vi "GetBarStartPosition.vi"(8 "error in (no error)":errorcluster, 11 "Code39 in":refnum<class "Code39.lvclass">) -> (0 "error out":errorcluster, 2 "Start Position":cluster{"x":i16, "y":i16}={"x"=10, "y"=3}, 3 "Code39 out":refnum<class "Code39.lvclass">)   [LabVIEW 2013, in "BarCodes.lvlib" / "Code39.lvclass"]
doc: "Specifies the top-left corner of the barcode in a given image. This effectively sets the quiet space in either direction around the bar code."
uses:
  Code39.lvclass
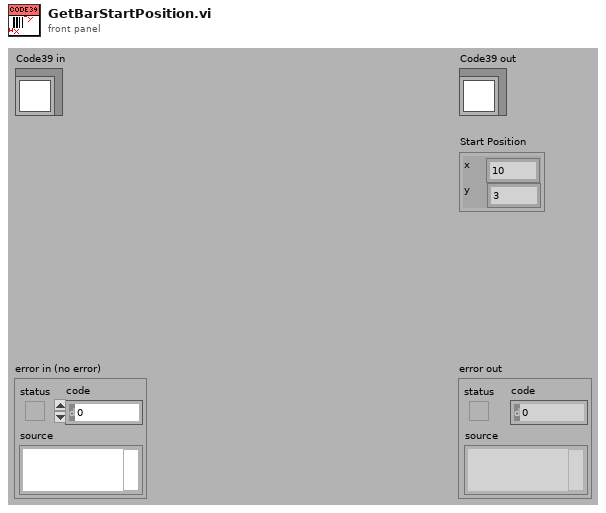
[diagram p1: front panel]
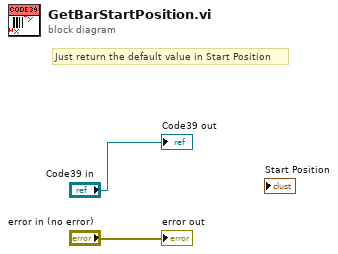
[diagram p0: block diagram]
diagram:
  # "Just return the default value in Start Position"
  "error out" <- "error in (no error)"
  "Code39 out" <- "Code39 in"
